vi "inspect lv class.vi"() -> ()   [LabVIEW 2023]
panel:
  out "Array":string[](array[string])
  out "error out":errorcluster
  in  "Path":path=path "C:/Program Files/National Instruments/LabVIEW 2023/user.lib/uhd/MultiUsrp/MultiUsrp.lvclass"
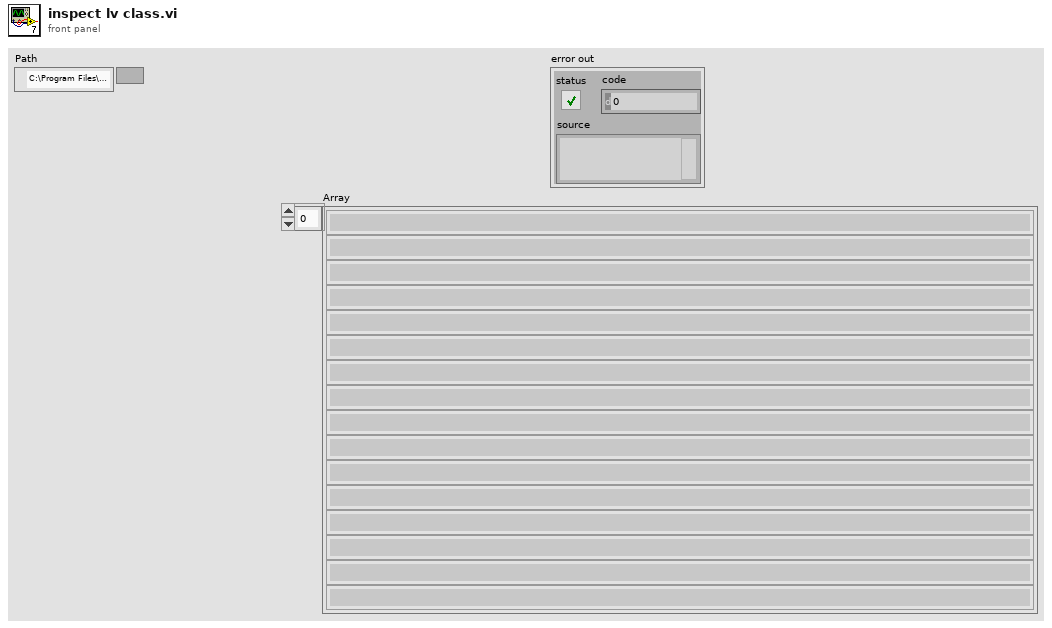
[diagram p1: front panel]
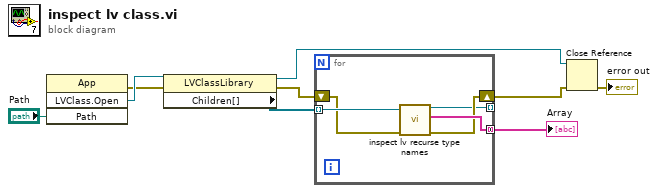
[diagram p0: block diagram]
diagram:
  n1 = invoke class="App" method="LVClass.Open"("Path"="Path") -> (error out=w6:errorcluster, "LVClass.Open"=w8:refnum<vi>)  [unwired: 3 in, 2 out]
  n2 = property class="LVClassLibrary"(reference=w8, error in=w6) -> (reference out=w3:refnum<vi>, error out=w5:errorcluster, "Children[]"=w7:refnum<vi>[])
  n3 = for {
    tunnel: w7 -> [w14] mode=indexing
    shift-right: [w11] -> w4
    shift-left: w5 -> [w12]
    tunnel: [w13] -> w1 mode=concatenating
    tunnel: [w10] -> _ mode=indexing
    n4 = call "inspect lv recurse type names.vi"("error in (no error)"=w12, "ProjectItem in"=w14) -> ("error out"=w11:errorcluster, "Type String"=w13:string[], "ProjectItem out"=w10:refnum<vi>)  [unwired: 7 in]
  }
  "Array" <- w1
  n5 = Close Reference(reference=w3, error in (no error)=w4) -> (error out=→"error out":errorcluster)
